vi "Chroma LabView.vi"() -> ()   [LabVIEW 2011]
uses:
  <vilib>/Utility/file.llb/Write To Spreadsheet File (string).vi
panel:
  in  "Name of File":string
  out "Current Data Point":i32
  in  "Interval of Data Collection (sec)":u32
  in  "Number of Data Points to Collect":i32
  in  "Type (P_REAL)":i32(ring) items=["P_ENERGY"=4, "P_FACTOR"=3, "P_REACTIVE"=2, "P_APPARENT"=1, "P_REAL"=0]
  in  "Type (I_RMS)":i32(ring) items=["I_THD"=5, "I_CRESTFACTOR"=4, "I_INRUSH"=3, "I_PEAK-"=2, "I_PEAK+"=1, "I_RMS"=0]
  in  "Type (V_RMS)":i32(ring) items=["V_THD"=3, "V_PEAK-"=2, "V_PEAK+"=1, "V_RMS"=0]
  in  "resource name 2":refnum<visa-resource-name> caption="resource name"
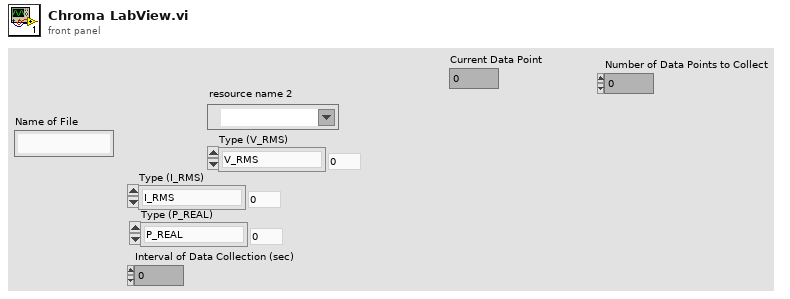
[diagram p1: front panel]
types:
  T1 = enum16{"open", "replace", "create", "open or create", "replace or create", "replace or create with confirmation"}
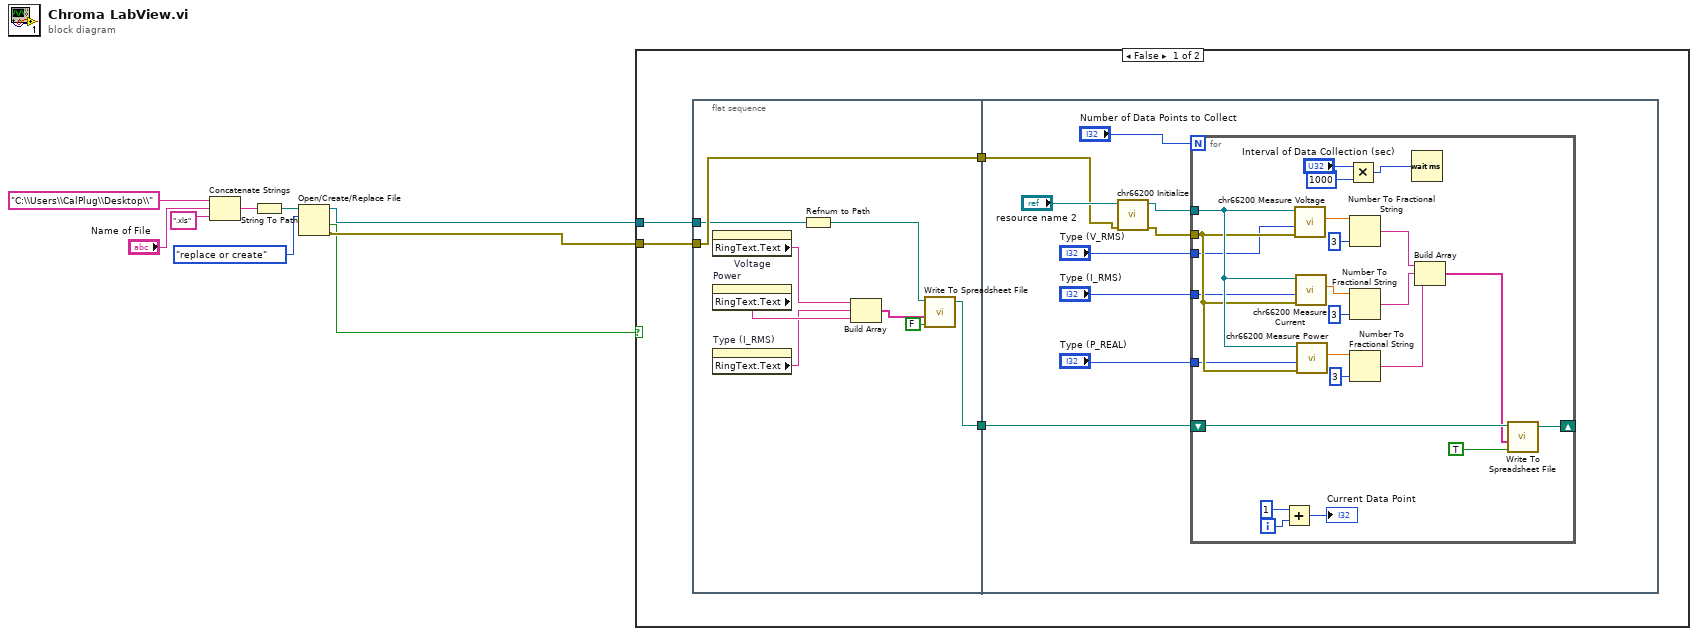
[diagram p0: block diagram]
diagram:
  n1 = Concatenate Strings("C:\\Users\\CalPlug\\Desktop\\" ("string"), "Name of File", ".xls" ("string")) -> (w9:string)
  n2 = String To Path(string=w9) -> (path=w8:path)
  n3 = Open/Create/Replace File(file path (use dialog)=w8, operation (0:open)=T1."replace or create") -> (refnum out=w2:refnum<file>, cancelled=w1:bool, error out=w3:errorcluster)  [unwired: 4 in]
  n4 = case shown="False" w1 {
    tunnel: w3 -> [w11 _]
    tunnel: w2 -> [w10 _]
    frame False {
      n5 = flat-sequence {
        tunnel: [w22] -> w13
        tunnel: [w19] -> w12
        tunnel: w11 -> [w19]
        tunnel: w10 -> [w14]
        tunnel: w13 -> [w24]
        tunnel: w12 -> [w23]
        frame #0 {
          n6 = property on="Voltage" class="Ring (strict)"() -> ("RingText.Text"=w18:string)  [unwired: 2 in, 2 out]
          n7 = property on="Power" class="Ring (strict)"() -> ("RingText.Text"=w17:string)  [unwired: 2 in, 2 out]
          n8 = property on="Type (I_RMS)" class="Ring (strict)"() -> ("RingText.Text"=w16:string)  [unwired: 2 in, 2 out]
          n9 = Refnum to Path(1:w14) -> (0:w20:path)
          n10 = Build Array(w18, w16, w17) -> (w15:string[])
          n11 = call-poly <vilib>:"Write To Spreadsheet File.vi"("append to file? (new file:F)"=FALSE, "1D data"=w15, "file path (dialog if empty)"=w20) -> ("new file path (Not A Path if cancelled)"=w22:path)  [unwired: 5 in]
        }
        frame #1 {
          n12 = call <instrlib>:"chr66200 Initialize.vi"("error in (no error)"=w23, "resource name"="resource name 2") -> ("error out"=w27:errorcluster, "instrument handle out"=w26:refnum<visa-resource-name>)  [unwired: 8 in]
          n13 = for {
            N: "Number of Data Points to Collect" -> [_]
            tunnel: w26 -> [w55]
            tunnel: w27 -> [w54]
            tunnel: "Type (I_RMS)" -> [w53]
            tunnel: "Type (V_RMS)" -> [w52]
            tunnel: "Type (P_REAL)" -> [w51]
            shift-right: [w49] -> _
            shift-left: w24 -> [w50]
            i -> [w40]
            n14 = Add(x=1, y=w40) -> (x+y=→"Current Data Point":i32)
            n15 = call <instrlib>:"chr66200 Measure Voltage.vi"("error in (no error)"=w54, "Type (V_RMS)"=w52, "instrument handle"=w55) -> ("Read Value"=w47:dbl)  [unwired: 6 in, 2 out]
            n16 = call <instrlib>:"chr66200 Measure Current.vi"("error in (no error)"=w54, "Type (I_RMS)"=w53, "instrument handle"=w55) -> ("Read Value"=w46:dbl)  [unwired: 6 in, 2 out]
            n17 = call <instrlib>:"chr66200 Measure Power.vi"("error in (no error)"=w54, "Type (P_REAL)"=w51, "instrument handle"=w55) -> ("Read Value"=w45:dbl)  [unwired: 6 in, 2 out]
            n18 = Multiply(x="Interval of Data Collection (sec)", y=u32 1000) -> (x*y=w35:u32)
            n19 = Number To Fractional String(number=w47, precision (6)=i16 3) -> (F-format string=w34:string)  [unwired: 2 in]
            n20 = Number To Fractional String(number=w46, precision (6)=i16 3) -> (F-format string=w33:string)  [unwired: 2 in]
            n21 = Number To Fractional String(number=w45, precision (6)=i16 3) -> (F-format string=w32:string)  [unwired: 2 in]
            n22 = Wait (ms)(milliseconds to wait=w35) -> ()  [unwired: 1 out]
            n23 = Build Array(w34, w33, w32) -> (w41:string[])
            n24 = call-poly <vilib>:"Write To Spreadsheet File.vi"("append to file? (new file:F)"=TRUE, "1D data"=w41, "file path (dialog if empty)"=w50) -> ("new file path (Not A Path if cancelled)"=w49:path)  [unwired: 5 in]
          }
        }
      }
    }
    frame True {
    }
  }
